vi "Assert False.vi"(7 "Message (\"\")":string, 8 "error in (no error)":errorcluster, 10 "Condition":bool) -> (0 "error out":errorcluster)   [LabVIEW 2017, in "Assertion.lvlib"]
doc: "Asserts that a condition is <B>false</B>. Does nothing if an error occurred before this node runs. Returns an error if the assertion failed. Optionally adds a message to the error message if the assertion failed."
uses:
  Assertion.lvlib
  Constraint/IsFalse/IsFalse.lvclass
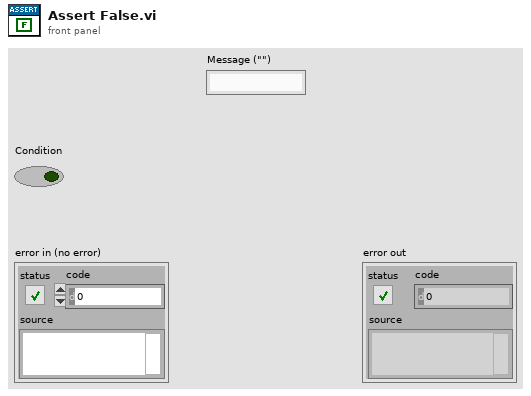
[diagram p1: front panel]
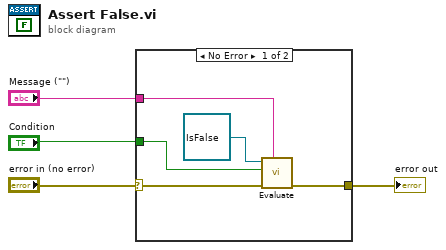
[diagram p0: block diagram]
diagram:
  n1 = case shown="No Error" "error in (no error)" {
    selector: "error in (no error)" -> [w8 w10]
    tunnel: "Condition" -> [w6 _]
    tunnel: [w7 w10] -> w1
    tunnel: "Message (\"\")" -> [w5 _]
    frame No Error {
      n2 = call-dynamic "Evaluate.vi"("Message (\"\")"=w5, "error in (no error)"=w8, "Actual"=w6, "Constraint in"=refnum<class "IsFalse.lvclass"> refnum ("IsFalse.lvclass")) -> ("error out"=w7:errorcluster)  [unwired: 6 in, 1 out]
    }
    frame Error {
    }
  }
  "error out" <- w1
